vi "Parse Tagged Packets From Disk.vi"(0 "llp tagged packet file path":path, 7 "packet start index":u64, 9 "num packets to read":i64=-1, 11 "error in":errorcluster, 12 "max bytes to read per iteration":i64=1048576) -> (4 "tagged packets":T1[](array[typedef]), 6 "total packets in file":i64, 8 "total tagged packet bytes in file":i64, 15 "error out":errorcluster)   [LabVIEW 2023, in "GettingStarted_Common_148X_Host.lvlib"]
uses:
  GettingStarted_Common_148X_Host.lvlib
  <instrlib>/FlexRIO/CSI-2/v2/Host/Types/Host Tagged LLP Packet.ctl
  <instrlib>/FlexRIO/CSI-2/v2/Host/Types/Host LLP Packet Tag.ctl
  <instrlib>/FlexRIO/CSI-2/v2/Host/Types/Host LLP Packet Timestamp.ctl
  <instrlib>/FlexRIO/CSI-2/v2/FPGA/Types/Timestamp ID.ctl
  <instrlib>/FlexRIO/CSI-2/v2/Host/Types/Host LLP Packet Size.ctl
  <instrlib>/FlexRIO/CSI-2/v2/Host/Types/Host LLP Packet.ctl
  <instrlib>/FlexRIO/CSI-2/v2/FPGA/Types/LLP Packet Header.ctl
  <instrlib>/FlexRIO/CSI-2/v2/FPGA/Types/LLP Packet Footer.ctl
  4c3d0605-e4fa-43fb-9214-80359bf2f300.vi
  <instrlib>/FlexRIO/CSI-2/v2/Host/NI CSI-2 API Host v2.lvlib
  <instrlib>/FlexRIO/CSI-2/v2/FPGA/NI CSI-2 API FPGA v2.lvlib
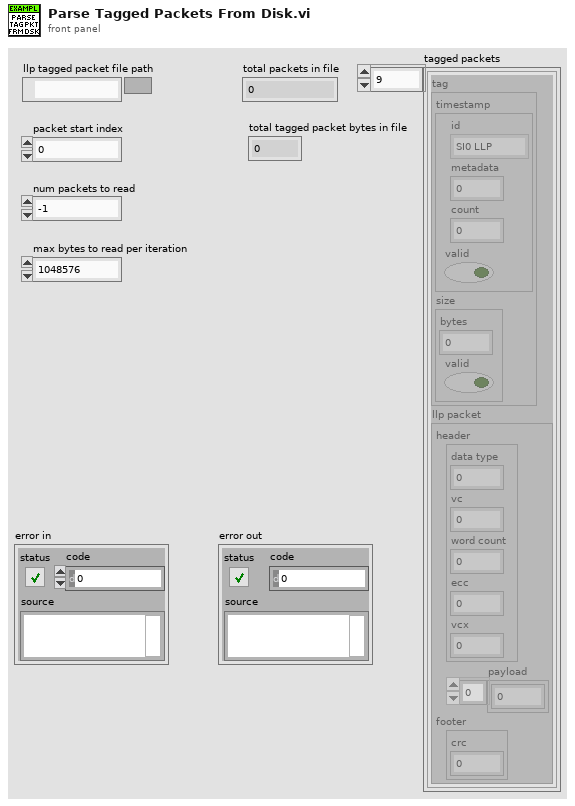
[diagram p1: front panel]
types:
  T1 = typedef "NI CSI-2 API Host v2.lvlib/Host Tagged LLP Packet.ctl" = cluster{"tag":T2, "llp packet":T6}
  T2 = typedef "NI CSI-2 API Host v2.lvlib/Host LLP Packet Tag.ctl" = cluster{"timestamp":T3, "size":T5}
  T3 = typedef "NI CSI-2 API Host v2.lvlib/Host LLP Packet Timestamp.ctl" = cluster{"valid":bool, "count":u64, "id":T4, "metadata":u8}
  T4 = typedef "NI CSI-2 API FPGA v2.lvlib/Timestamp ID.ctl" = enum8{"SI0 LLP", "SI1 LLP", "SI2 LLP", "SI3 LLP", "SI4 LLP", "SI5 LLP", "SI6 LLP", "SI7 LLP", "SO0 LLP", "SO1 LLP", "SO2 LLP", "SO3 LLP", "SO4 LLP", "SO5 LLP", "SO6 LLP", "SO7 LLP", "Ser0 GPIO Bank", "Ser1 GPIO Bank", "Ser2 GPIO Bank", "Ser3 GPIO Bank", "Ser4 GPIO Bank", "Ser5 GPIO Bank", "Ser6 GPIO Bank", "Ser7 GPIO Bank", "Des0 GPIO Bank", "Des1 GPIO Bank", "Des2 GPIO Bank", "Des3 GPIO Bank", "Des4 GPIO Bank", "Des5 GPIO Bank", "Des6 GPIO Bank", "Des7 GPIO Bank", "User0", "User1", "User2", "User3", "User4", "User5", "User6", "User7", "User8", "User9", "User10", "User11", "User12", "User13", "User14", "User15", "User16", "User17", "User18", "User19", "User20", "User21", "User22", "User23", "User24", "User25", "User26", "User27", "User28", "User29", "User30", "User31"}
  T5 = typedef "NI CSI-2 API Host v2.lvlib/Host LLP Packet Size.ctl" = cluster{"bytes":u32, "valid":bool}
  T6 = typedef "NI CSI-2 API Host v2.lvlib/Host LLP Packet.ctl" = cluster{"header":T7, "payload":u8[], "footer":T8}
  T7 = typedef "NI CSI-2 API FPGA v2.lvlib/LLP Packet Header.ctl" = cluster{"word count":u16, "ecc":fxp<+,6,6>, "vcx":fxp<+,2,2>, "data type":fxp<+,6,6>, "vc":fxp<+,2,2>}
  T8 = typedef "NI CSI-2 API FPGA v2.lvlib/LLP Packet Footer.ctl" = cluster{"crc":u16}
  T9 = enum16{"open", "open or create", "create or replace", "create", "open (read-only)"}
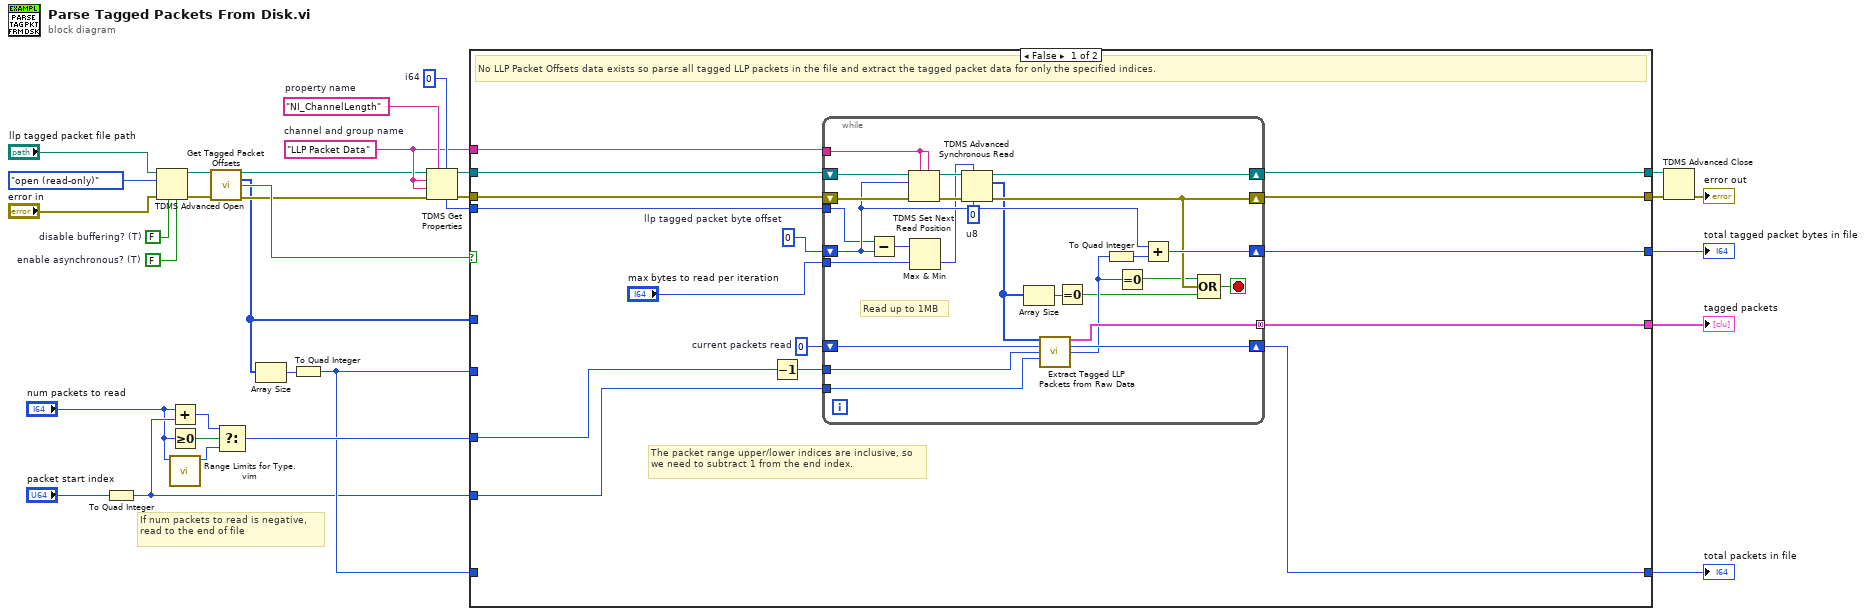
[diagram p0: block diagram]
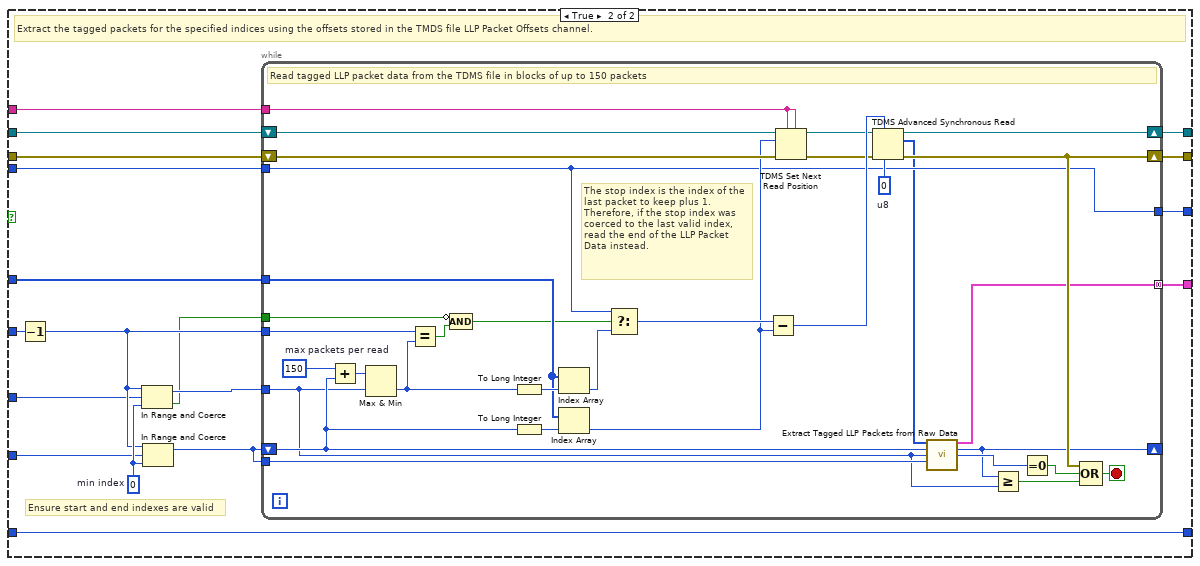
[diagram p2: hidden frame]
diagram:
  w17 = i64 0  # i64
  w16 = "NI_ChannelLength"  # property name
  w14 = "LLP Packet Data"  # channel and group name
  w29 = FALSE  # disable buffering? (T)
  w32 = FALSE  # enable asynchronous? (T)
  # "If num packets to read is negative, read to the end of file"
  n1 = To Quad Integer(1:"packet start index") -> (0:w3:i64)
  n2 = TDMS Advanced Open(4:w32, 6:w29, 8:"error in", 10:T9."open (read-only)" ("operation (0:open)"), 11:"llp tagged packet file path") -> (0:w18:errorcluster, 3:w19:refnum<k34>)  [unwired: 1 out]
  n3 = Add(x="num packets to read", y=w3) -> (x+y=w1:i64)
  n4 = Greater Or Equal To 0?(x="num packets to read") -> (x >= 0?=w26:bool)
  n5 = call "Range Limits for Type.vim"("type"="num packets to read") -> ("maximum value for type"=w25:i64)  [unwired: 9 in, 1 out]
  n6 = call "Get Tagged Packet Offsets.vi"("tdms file in"=w19, "error in"=w18) -> ("tdms file out"=w9:refnum<k34>, "tagged packet offsets"=w6:i64[], "packet offsets valid?"=w10:bool, "error out"=w8:errorcluster)  [unwired: 10 in]
  n7 = Select(t=w1, s=w26, f=w25) -> (s? t:f=w24:i64)
  n8 = Array Size(array=w6) -> (size(s)=w5:i32)
  n9 = To Quad Integer(1:w5) -> (0:w4:i64)
  n10 = TDMS Get Properties(5:w17, 7:w16, 8:w8, 9:w14, 10:w14, 11:w9) -> (0:w13:errorcluster, 3:w12:refnum<k34>, 4:w15:i64)  [unwired: 3 out]
  n11 = case shown="False" w10 {
    tunnel: [w47 w77] -> w31
    tunnel: [w46 w80] -> w30
    tunnel: w24 -> [w34 w74]
    tunnel: [w35 w78] -> w22
    tunnel: [w43 w79] -> w21
    tunnel: w3 -> [w42 w85]
    tunnel: [w41 w76] -> w20
    tunnel: w6 -> [_ w90]
    tunnel: w15 -> [w40 w88]
    tunnel: w14 -> [w39 w82]
    tunnel: w13 -> [w38 w83]
    tunnel: w12 -> [w37 w84]
    tunnel: w4 -> [_ w89]
    tunnel: w4 -> [_ w78]
    frame False {
      w44 = i64 0  # current packets read
      w45 = i64 0  # llp tagged packet byte offset
      # "The packet range upper/lower indices are inclusive, so we need to subtract 1 from the end index."
      # "No LLP Packet Offsets data exists so parse all tagged LLP packets in the file and extract the tagged packet data for only the specified indices."
      n12 = Decrement(x=w34) -> (x-1=w33:i64)
      n13 = while {
        shift-right: [w65] -> w46
        shift-left: w38 -> [w72]
        shift-right: [w49] -> w47
        shift-left: w37 -> [w71]
        shift-right: [w69] -> w41
        shift-left: w45 -> [w63]
        tunnel: "max bytes to read per iteration" -> [w61]
        tunnel: w42 -> [w56]
        tunnel: [w54] -> w43 mode=concatenating
        shift-right: [w53] -> w35
        shift-left: w44 -> [w55]
        tunnel: w40 -> [w59]
        tunnel: w39 -> [w58]
        tunnel: w33 -> [w48]
        stop <- w67 stop-if-true
        w73 = u8 0  # u8
        # "Read up to 1MB"
        n14 = Subtract(x=w59, y=w63) -> (x-y=w62:i64)
        n15 = TDMS Set Next Read Position(5:w58, 7:w58, 8:w72, 10:w63, 11:w71) -> (0:w68:errorcluster, 3:w70:refnum<k34>)  [unwired: 1 in]
        n16 = Max & Min(x=w62, y=w61) -> (min(x,y)=w60:i64)  [unwired: 1 out]
        n17 = TDMS Advanced Synchronous Read(6:w73, 7:w60, 8:w68, 11:w70) -> (0:w65:errorcluster, 2:w57:u8[], 3:w49:refnum<k34>)  [unwired: 1 out]
        n18 = Array Size(array=w57) -> (size(s)=w64:i32)
        n19 = call "Extract Tagged LLP Packets from Raw Data.vi"("tagged packet data block"=w57, "block start packet index"=w55, "packet range upper"=w48, "packet range lower"=w56) -> ("tagged packets"=w54:T1[], "block end packet index"=w53:i64, "block bytes parsed"=w52:u32)  [unwired: 9 in]
        n20 = Equal To 0?(x=w64) -> (x = 0?=w50:bool)
        n21 = To Quad Integer(1:w52) -> (0:w66:i64)
        n22 = Equal To 0?(x=w52) -> (x = 0?=w51:bool)
        n23 = Add(x=w63, y=w66) -> (x+y=w69:i64)
        n24 = Compound Arithmetic op=OR(w51, w65, w50) -> (w67:bool)
      }
    }
    frame True {
      w91 = i64 0  # min index
      # "Ensure start and end indexes are valid"
      # "Extract the tagged packets for the specified indices using the offsets stored in the TMDS file LLP Packet Offsets channel."
      n25 = Decrement(x=w89) -> (x-1=w86:i64)
      n26 = In Range and Coerce(upper limit=w86, x=w74, lower limit=w91) -> (coerced(x)=w87:i64, In Range?=w81:bool)
      n27 = In Range and Coerce(upper limit=w86, x=w85, lower limit=w91) -> (coerced(x)=w75:i64)  [unwired: 1 out]
      n28 = while {
        tunnel: w87 -> [w96]
        tunnel: w90 -> [w122]
        tunnel: w88 -> [w104]
        shift-right: [w93] -> _
        shift-left: w75 -> [w99]
        tunnel: w86 -> [w117]
        tunnel: w82 -> [w114]
        tunnel: w81 -> [w102]
        shift-right: [w106] -> w80
        shift-left: w83 -> [w115]
        tunnel: [w92] -> w79 mode=concatenating
        shift-right: [w108] -> w77
        shift-left: w84 -> [w116]
        tunnel: [w104] -> w76
        tunnel: w75 -> [w98]
        stop <- w107 stop-if-true
        w109 = u8 0  # u8
        w118 = i64 150  # max packets per read
        # "The stop index is the index of the last packet to keep plus 1.  Therefore, if the stop index was coerced to the last valid index, read the end of the LLP Packet Data instead."
        # "Read tagged LLP packet data from the TDMS file in blocks of up to 150 packets"
        n29 = Add(x=w118, y=w99) -> (x+y=w121:i64)
        n30 = Max & Min(x=w121, y=w96) -> (min(x,y)=w100:i64)  [unwired: 1 out]
        n31 = Equal?(x=w117, y=w100) -> (x = y?=w101:bool)
        n32 = Compound Arithmetic op=AND(invert w102, w101) -> (w103:bool)
        n33 = To Long Integer(number=w100) -> (32bit integer=w124:i32)
        n34 = To Long Integer(number=w99) -> (32bit integer=w123:i32)
        n35 = Index Array(array=w122, index=w124) -> (element=w120:i64)
        n36 = Index Array(array=w122, index=w123) -> (element=w113:i64)
        n37 = Select(t=w104, s=w103, f=w120) -> (s? t:f=w119:i64)
        n38 = Subtract(x=w119, y=w113) -> (x-y=w112:i64)
        n39 = TDMS Set Next Read Position(5:w114, 7:w114, 8:w115, 10:w113, 11:w116) -> (0:w111:errorcluster, 3:w110:refnum<k34>)  [unwired: 1 in]
        n40 = TDMS Advanced Synchronous Read(6:w109, 7:w112, 8:w111, 11:w110) -> (0:w106:errorcluster, 2:w97:u8[], 3:w108:refnum<k34>)  [unwired: 1 out]
        n41 = call "Extract Tagged LLP Packets from Raw Data.vi"("tagged packet data block"=w97, "block start packet index"=w99, "packet range upper"=w96, "packet range lower"=w98) -> ("tagged packets"=w92:T1[], "block end packet index"=w93:i64, "block bytes parsed"=w94:u32)  [unwired: 9 in]
        n42 = Greater Or Equal?(x=w93, y=w96) -> (x >= y?=w95:bool)
        n43 = Equal To 0?(x=w94) -> (x = 0?=w105:bool)
        n44 = Compound Arithmetic op=OR(w106, w105, w95) -> (w107:bool)
      }
    }
  }
  "total packets in file" <- w22
  "tagged packets" <- w21
  "total tagged packet bytes in file" <- w20
  n45 = TDMS Advanced Close(8:w30, 11:w31) -> (0:→"error out":errorcluster)  [unwired: 2 in, 1 out]
